vi "App_Queue.vi"(7 "Error_Connection":refnum<vi>, 8 "error in":errorcluster) -> (0 "error out":errorcluster, 3 "Queues out":T1, 5 "Error Conneciton":bool)   [LabVIEW 2019]
uses:
  TypeDef/#TypeDef_App_Queues.ctl
  User Interface/TypeDef/#TypeDef_Enum_Buttons.ctl
  User Interface/TypeDef/#TypeDef_EventStructureConstant.ctl
  User Interface/TypeDef/#TypeDef_Enum_EventStructure.ctl
  TypeDef/#TypeDef_NetworkStream.ctl
  Communication/TypeDef/#TypeDef_FromMRtoPC.ctl
  Communication/TypeDef/#TypeDef_FromPCtoMR.ctl
  Communication/TypeDef/#TypeDef_Command.ctl
  Communication/TypeDef/#TypeDef_ErrorHandler_prop.ctl
  Communication/TypeDef/#TypeDef_PropGraph.ctl
  Communication/TypeDef/#TypeDef_PropertiesToSave.ctl
  <vilib>/addons/database/Connection.llb/Conn ObjectReference.ctl
  Test/TypeDef/#TypeDef_DataToTest.ctl
  Communication/TypeDef/#TypeDef_EnumConnection.ctl
  <vilib>/addons/database/NI_Database_API.lvlib
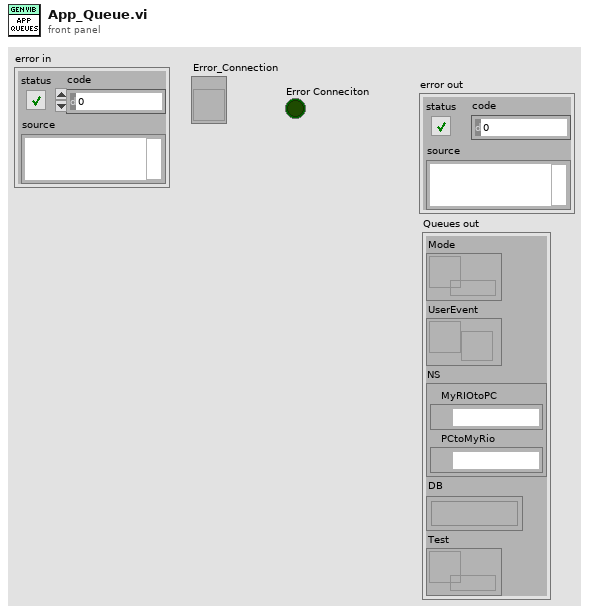
[diagram p1: front panel]
types:
  T1 = typedef "#TypeDef_App_Queues.ctl" = cluster{"Mode":refnum<queue>, "UserEvent":refnum<user-event>, "NS":T2, "DB":T3, "Test":refnum<queue>}
  T2 = typedef "#TypeDef_NetworkStream.ctl" = cluster{"MyRIOtoPC":refnum<k21>, "PCtoMyRio":refnum<k21>}
  T3 = typedef "NI_Database_API.lvlib/Conn ObjectReference.ctl" = refnum<k1>
  T4 = typedef "#TypeDef_EnumConnection.ctl" = enum16{"Try to Connect PCMyRio", "Try to Connect MyRioPC", "Send queues", "Error"}
  T5 = typedef "#TypeDef_FromPCtoMR.ctl" = cluster{"Command":T6, "Error?":bool, "Stop":bool, "StopPomiar":bool, "Name":string, "FilesPath":path, "ErrorHandler":T7, "Fs":dbl}
  T6 = typedef "#TypeDef_Command.ctl" = enum16{"Start", "End"}
  T7 = typedef "#TypeDef_ErrorHandler_prop.ctl" = cluster{"Threads":enum16{"Acquisistion", "Data Operation", "Save File"}, "ClearError":bool, "Error Out ":errorcluster, "Error":bool}
  T8 = typedef "#TypeDef_FromMRtoPC.ctl" = cluster{"Accessibility":T5, "PropGraph":T9, "No Data?":bool, "WaveformData":waveform(dbl)[]}
  T9 = typedef "#TypeDef_PropGraph.ctl" = cluster{"Raw Data":dbl[][], "Poperties":T10, "Power Spectrum / PSD":cluster{"f0":dbl, "df":dbl, "magnitude":dbl[]}[]}
  T10 = typedef "#TypeDef_PropertiesToSave.ctl" = cluster{"RMS values":dbl[], "Max":dbl[], "Min":dbl[], "A(8)":dbl[], "t":dbl, "A(8) Axis":dbl, "Aw":dbl[], "Ak 30min":dbl, "Ak_axis":i32, "Spec":cluster{"f0":dbl, "df":dbl, "magnitude":dbl[]}[]}
  T11 = typedef "#TypeDef_DataToTest.ctl" = cluster{"FilesPath":path, "Name_Meas":string, "stop":bool, "Command":T6, "Fs":dbl, "Test":bool}
  T12 = typedef "#TypeDef_Enum_Buttons.ctl" = enum32{"MainPage", "Pomiar", "Archiwum", "Operacje", "Wyjœcie"}
  T13 = typedef "#TypeDef_EventStructureConstant.ctl" = cluster{"Value":variant, "Property":T14}
  T14 = typedef "#TypeDef_Enum_EventStructure.ctl" = enum16{"Default", "Final Items", "Moment Items", "DB"}
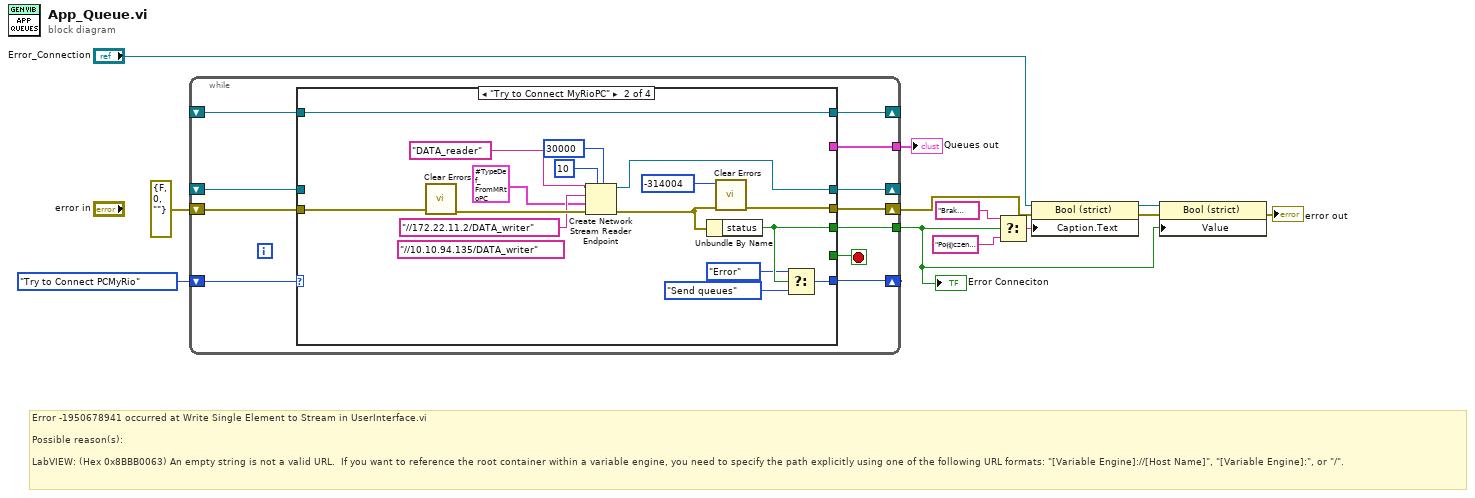
[diagram p0: block diagram]
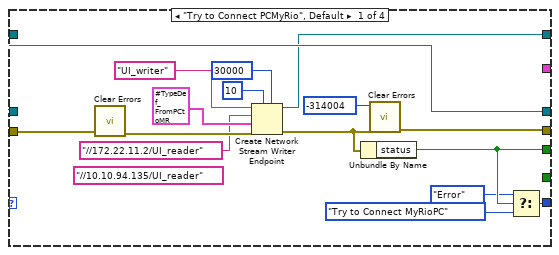
[diagram p2: hidden frame]
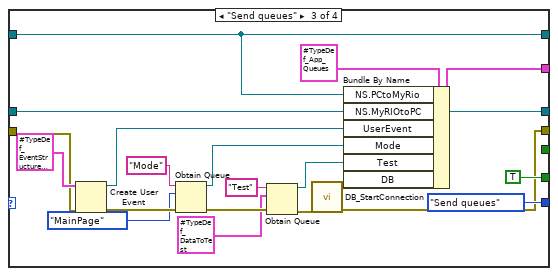
[diagram p3: hidden frame]
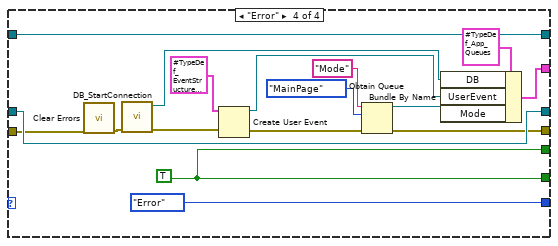
[diagram p4: hidden frame]
diagram:
  # "Error -1950678941 occurred at Write Single Element to Stream in UserInterface.vi\n\nPossible reason(s):\n\nLabVIEW: (Hex 0x8BBB0063) An empty string is not a valid URL.  If you want to reference the root container within a variable engine, you need to specify the path explicitly using one of the following URL formats: \"[Variable Engine]://[Host Name]\", \"[Variable Engine]:\", or \"/\"."
  n1 = while {
    shift-right: [w23] -> w6
    shift-left: errorcluster {"status"=FALSE, "code"=0, "source"=""} ("error out") -> [w22]
    shift-right: [w21] -> _
    shift-left: _ -> [w14]
    shift-right: [w20] -> _
    shift-left: _ -> [w15]
    shift-right: [w17] -> _
    shift-left: #TypeDef_EnumConnection."Try to Connect PCMyRio" -> [w16]
    tunnel: [w18] -> w3
    tunnel: [w13] -> w1
    stop <- w19 stop-if-true
    n2 = case shown="\"Try to Connect MyRioPC\"" w16 {
      tunnel: [w33 w51 w71 w80] -> w23
      tunnel: w22 -> [w29 w45 w62 w79]
      tunnel: [w27 w49 w73 w91] -> w21
      tunnel: [w35 w43 w72 w90] -> w20
      tunnel: w14 -> [_ w49 w73 w91]
      tunnel: w15 -> [w35 _ w72 w90]
      tunnel: [_ _ TRUE w92] -> w19
      tunnel: [w34 w50 _ w92] -> w18
      tunnel: [w38 w54 #TypeDef_EnumConnection."Send queues" #TypeDef_EnumConnection."Error"] -> w17
      tunnel: [_ _ w61 w83] -> w13
      frame "Try to Connect PCMyRio", Default {
        (unwired) "//10.10.94.135/UI_reader"
        n3 = call <vilib>:"Clear Errors.vi"("error in (no error)"=w29) -> ("error out"=w28:errorcluster)  [unwired: 5 in, 1 out]
        n4 = Create Network Stream Writer Endpoint(5:30000 ("timeout in ms (-1)"), 7:10 ("writer buffer size"), 8:w28, 9:T5 {"Command"=enum."End", "Error?"=FALSE, "Stop"=FALSE, "StopPomiar"=FALSE, "Name"="", "FilesPath"=path "", "ErrorHandler"={"Threads"=enum."Acquisistion", "ClearError"=FALSE, "Error Out "={"status"=FALSE, "code"=0, "source"=""}, "Error"=FALSE}, "Fs"=0.0} ("PCtoMyRio"), 10:"//172.22.11.2/UI_reader", 11:"UI_writer" ("writer name")) -> (0:w39:errorcluster, 3:w27:refnum<k21>)  [unwired: 1 in]
        n5 = Unbundle By Name(w39) -> ("status"=w34:bool)
        n6 = call <vilib>:"Clear Errors.vi"("error in (no error)"=w39, "specific error code to clear (0: all)"=-314004) -> ("error out"=w33:errorcluster)  [unwired: 4 in, 1 out]
        n7 = Select(t=#TypeDef_EnumConnection."Error", s=w34, f=#TypeDef_EnumConnection."Try to Connect MyRioPC") -> (s? t:f=w38:T4)
      }
      frame "Try to Connect MyRioPC" {
        (unwired) "//10.10.94.135/DATA_writer"
        n8 = call <vilib>:"Clear Errors.vi"("error in (no error)"=w45) -> ("error out"=w44:errorcluster)  [unwired: 5 in, 1 out]
        n9 = Create Network Stream Reader Endpoint(5:30000 ("timeout in ms (-1)"), 7:10 ("writer buffer size"), 8:w44, 9:T8 {"Accessibility"={"Command"=enum."End", "Error?"=FALSE, "Stop"=FALSE, "StopPomiar"=FALSE, "Name"="", "FilesPath"=path "", "ErrorHandler"={"Threads"=enum."Acquisistion", "ClearError"=FALSE, "Error Out "={"status"=FALSE, "code"=0, "source"=""}, "Error"=FALSE}, "Fs"=0.0}, "PropGraph"={"Raw Data"=[[0.0], [0.0234375], [0.9609375]], "Poperties"={"RMS values"=[], "Max"=[], "Min"=[], "A(8)"=[], "t"=0.0, "A(8) Axis"=0.0, "Aw"=[], "Ak 30min"=0.0, "Ak_axis"=0, "Spec"=[]}, "Power Spectrum / PSD"=[]}, "No Data?"=FALSE, "WaveformData"=[]} ("FromMyRiOtoUI"), 10:"//172.22.11.2/DATA_writer", 11:"DATA_reader" ("writer name")) -> (0:w55:errorcluster, 3:w43:refnum<k21>)  [unwired: 1 in]
        n10 = Unbundle By Name(w55) -> ("status"=w50:bool)
        n11 = call <vilib>:"Clear Errors.vi"("error in (no error)"=w55, "specific error code to clear (0: all)"=-314004) -> ("error out"=w51:errorcluster)  [unwired: 4 in, 1 out]
        n12 = Select(t=#TypeDef_EnumConnection."Error", s=w50, f=#TypeDef_EnumConnection."Send queues") -> (s? t:f=w54:T4)
      }
      frame "Send queues" {
        n13 = Create User Event(user event datatype=T13 {"Value"=variant, "Property"=enum."Default"} ("EventStr"), error in=w62) -> (user event=w67:refnum<user-event>, error out=w69:errorcluster)
        n14 = Obtain Queue(name (unnamed)="Mode", element data type=#TypeDef_Enum_Buttons."MainPage" ("Value"), error in (no error)=w69) -> (queue out=w66:refnum<queue>, error out=w60:errorcluster)  [unwired: 2 in, 1 out]
        n15 = Obtain Queue(name (unnamed)="Test", element data type=T11 {"FilesPath"=path "", "Name_Meas"="", "stop"=FALSE, "Command"=enum."Start", "Fs"=1000.0, "Test"=FALSE}, error in (no error)=w60) -> (queue out=w56:refnum<queue>, error out=w59:errorcluster)  [unwired: 2 in, 1 out]
        n16 = call "DB_StartConnection.vi"("error in (no error)"=w59) -> ("error out"=w71:errorcluster, "Refnum out"=w63:T3)  [unwired: 9 in]
        n17 = Bundle By Name(cluster=T1 {"Mode"=refnum, "UserEvent"=refnum, "NS"={"MyRIOtoPC"="", "PCtoMyRio"=""}, "DB"=refnum, "Test"=refnum} ("App_Queues"), "NS.PCtoMyRio"=w73, "NS.MyRIOtoPC"=w72, "UserEvent"=w67, "Mode"=w66, "Test"=w56, "DB"=w63) -> (w61:T1)
      }
      frame "Error" {
        w92 = TRUE
        n18 = call <vilib>:"Clear Errors.vi"("error in (no error)"=w79) -> ("error out"=w78:errorcluster)  [unwired: 5 in, 1 out]
        n19 = call "DB_StartConnection.vi"("error in (no error)"=w78) -> ("error out"=w77:errorcluster, "Refnum out"=w76:T3)  [unwired: 9 in]
        n20 = Create User Event(user event datatype=T13 {"Value"=variant, "Property"=enum."Default"} ("EventStr"), error in=w77) -> (user event=w82:refnum<user-event>, error out=w85:errorcluster)
        n21 = Obtain Queue(name (unnamed)="Mode", element data type=#TypeDef_Enum_Buttons."MainPage" ("Value"), error in (no error)=w85) -> (queue out=w81:refnum<queue>, error out=w80:errorcluster)  [unwired: 2 in, 1 out]
        n22 = Bundle By Name(cluster=T1 {"Mode"=refnum, "UserEvent"=refnum, "NS"={"MyRIOtoPC"="", "PCtoMyRio"=""}, "DB"=refnum, "Test"=refnum} ("App_Queues"), "DB"=w76, "UserEvent"=w82, "Mode"=w81) -> (w83:T1)
      }
    }
  }
  "Error Conneciton" <- w3
  "Queues out" <- w1
  n23 = Select(t="Brak po彻czenia z MyRio", s=w3, f="Po彻czenie z MyRio") -> (s? t:f=w9:string)
  n24 = property class="Bool (strict)"(reference="Error_Connection", error in=w6, "Caption.Text"=w9) -> (reference out=w4:refnum<vi>, error out=w5:errorcluster)
  n25 = property class="Bool (strict)"(reference=w4, error in=w5, "Value"=w3) -> (error out=→"error out":errorcluster)  [unwired: 1 out]
